vi "(B) Strain Calibration (SubVI).vi"(0 "References":T1, 9 "Strain Input":T3={"cDAQ Chassis"=1, "9237 Slot"=1, "Signals"=[0.10457461685625713, 0.10457461685625713, 0.10457461685625713, 0.10457461685625713]}) -> (6 "Strain OK?":bool, 8 "Strain Values":T2={"Output Values"=[1.9176191262786784, -5.904090522496145, 9.846069970789538, 2.5400406567394125], "Linear Equations"=[["f(x) = 18.337(x)+(0.000)", "18.337", "0.000"], ["f(x) = 22.199(x)+(-8.225)", "22.199", "-8.225"], ["f(x) = 94.154(x)+(0.000)", "94.154", "0.000"], ["f(x) = 24.289(x)+(0.000)", "24.289", "0.000"]], "COF Values"=[0.0, 0.0, 0.0, 0.0], "Signals"=[0.10457461685625713, 0.10457461685625713, 0.10457461685625713, 0.10457461685625713]}, 15 "Calibration Error":errorcluster)   [LabVIEW 2010]
panel:
  in  "Simulation":T4
  in  "Error Input":errorcluster
  in  "Calibration":T5={"Set?"=[FALSE, FALSE, FALSE, FALSE, FALSE, FALSE, FALSE, FALSE], "HI/LO Setpoints"=[10.0, 0.0, 10.0, 0.0, 10.0, 0.0, 10.0, 0.0], "HI/LO Signals"=[1.0, 0.0, 1.0, 0.0, 1.0, 0.0, 1.0, 0.0], "IN/OUT Signals"=[1.0, 0.0, 1.0, 0.0, 1.0, 0.0, 1.0, 0.0]} {"IN/OUT Signals" step=0.001 format="%#_4p"; "HI/LO Signals" step=0.001 format="%#_4p"; "HI/LO Setpoints" step=0.001 format="%#.2p"}
  # "Set\nValues?"
  # "Setpoint\nValues"
  # "Saved\nSignals"
  # "Calibration\nResult"
  # "Ch."
  # "IN"
  # "HI"
  # "0"
  # "LO"
  # "OUT"
  # "IN"
  # "HI"
  # "3"
  # "LO"
  # "OUT"
  # "IN"
  # "HI"
  # "2"
  # "LO"
  # "OUT"
  # "IN"
  # "HI"
  # "1"
  # "LO"
  # "OUT"
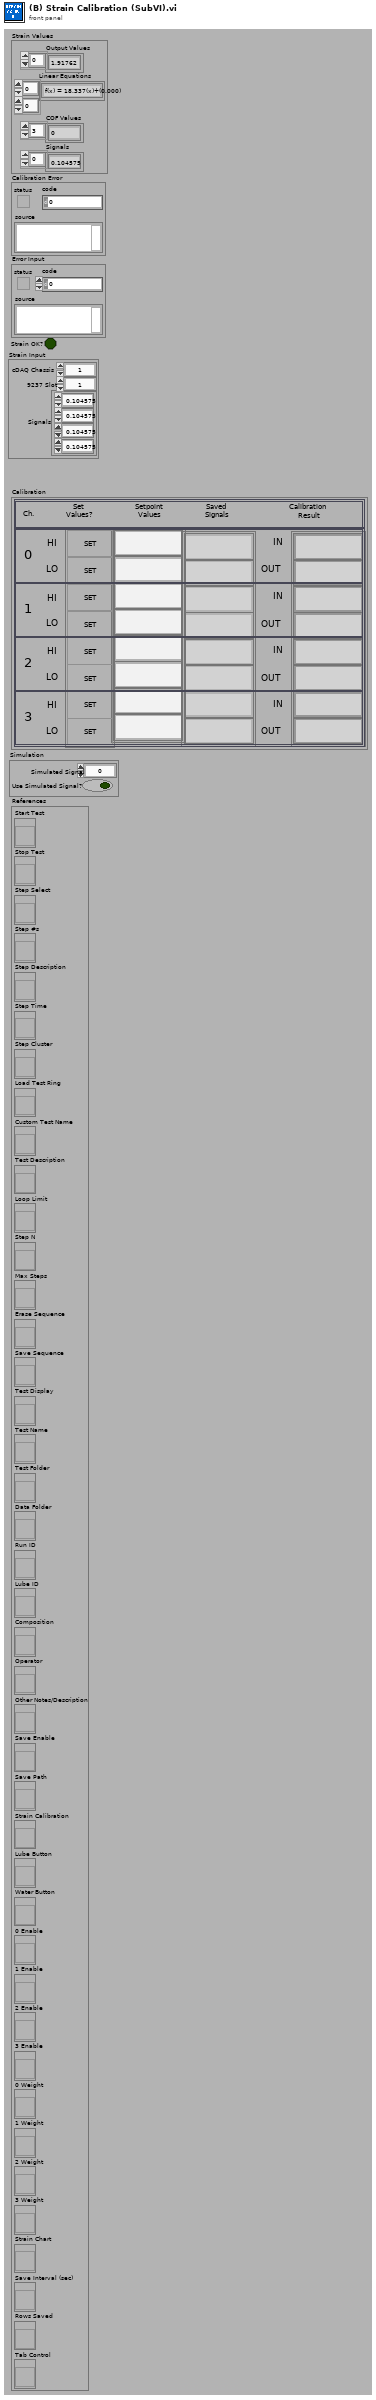
[diagram p1: front panel]
types:
  T1 = cluster{"Start Test":refnum<vi>, "Stop Test":refnum<vi>, "Step Select":refnum<vi>, "Step #s":refnum<vi>, "Step Description":refnum<vi>, "Step Time":refnum<vi>, "Step Cluster":refnum<vi>, "Load Test Ring":refnum<vi>, "Custom Test Name":refnum<vi>, "Test Description":refnum<vi>, "Loop Limit":refnum<vi>, "Step N":refnum<vi>, "Max Steps":refnum<vi>, "Erase Sequence":refnum<vi>, "Save Sequence":refnum<vi>, "Test Display":refnum<vi>, "Test Name":refnum<vi>, "Test Folder":refnum<vi>, "Data Folder":refnum<vi>, "Run ID":refnum<vi>, "Lube ID":refnum<vi>, "Composition":refnum<vi>, "Operator":refnum<vi>, "Other Notes/Description":refnum<vi>, "Save Enable":refnum<vi>, "Save Path":refnum<vi>, "Strain Calibration":refnum<vi>, "Lube Button":refnum<vi>, "Water Button":refnum<vi>, "0 Enable":refnum<vi>, "1 Enable":refnum<vi>, "2 Enable":refnum<vi>, "3 Enable":refnum<vi>, "0 Weight":refnum<vi>, "1 Weight":refnum<vi>, "2 Weight":refnum<vi>, "3 Weight":refnum<vi>, "Strain Chart":refnum<vi>, "Save Interval (sec)":refnum<vi>, "Rows Saved":refnum<vi>, "Tab Control":refnum<vi>}
  T2 = cluster{"Output Values":dbl[], "Linear Equations":string[][], "COF Values":dbl[], "Signals":dbl[]}
  T3 = cluster{"cDAQ Chassis":i32, "9237 Slot":i32, "Signals":dbl[]}
  T4 = cluster{"Use Simulated Signal?":bool, "Simulated Signal":dbl}
  T5 = cluster{"Set?":bool[], "HI/LO Setpoints":dbl[], "HI/LO Signals":dbl[], "IN/OUT Signals":dbl[]}
  T6 = enum16{"open", "replace", "create", "open or create", "replace or create", "replace or create with confirmation"}
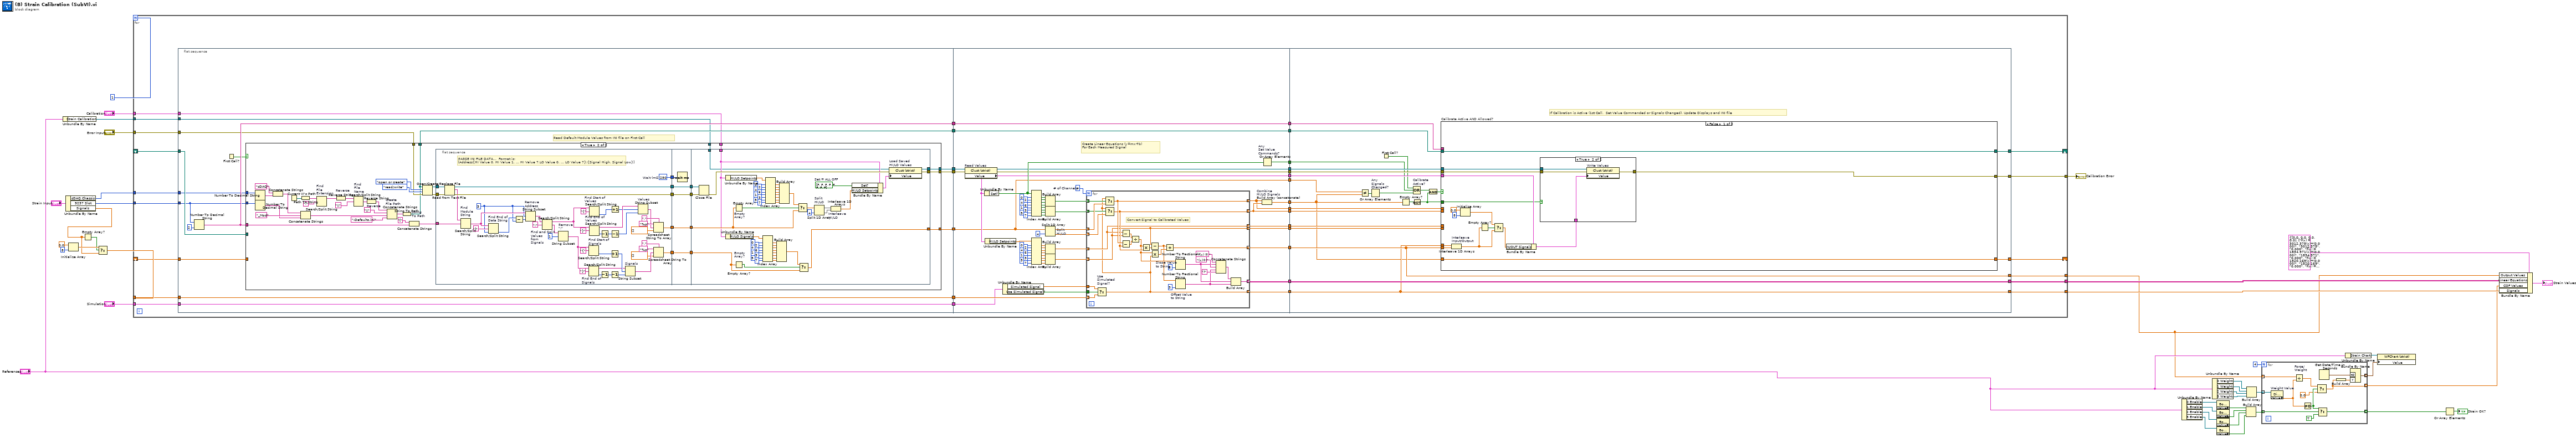
[diagram p0: block diagram]
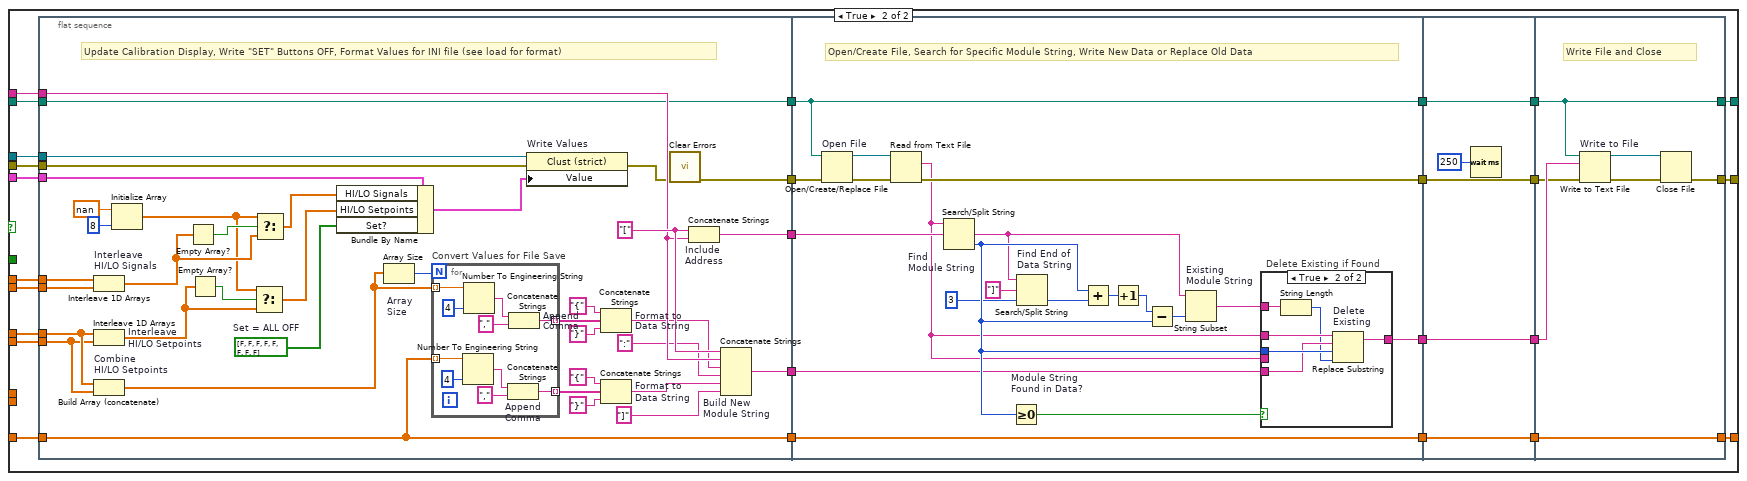
[diagram p4: hidden frame]
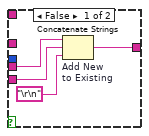
[diagram p5: hidden frame]
diagram:
  n1 = Unbundle By Name("References") -> ("Strain Calibration"=w24:refnum<vi>)
  n2 = Unbundle By Name("Strain Input") -> ("cDAQ Chassis"=w36:i32, "9237 Slot"=w37:i32, "Signals"=w8:dbl[])
  n3 = Initialize Array(0.0, 8) -> (w10:dbl[])
  n4 = Empty Array?(array=w8) -> (empty?=w9:bool)
  n5 = Select(t=w10, s=w9, f=w8) -> (s? t:f=w7:dbl[])
  n6 = for {
    N: 1 -> [_]
    shift-right: [w77] -> _
    shift-left: _ -> [w78]
    tunnel: [w76] -> w13
    shift-right: [w73] -> _
    shift-left: _ -> [w72]
    tunnel: w24 -> [w42]
    tunnel: [w75] -> w1
    tunnel: [w74] -> w27
    tunnel: "Error Input" -> [w67]
    tunnel: [w65] -> w28
    tunnel: "Calibration" -> [w64]
    tunnel: w36 -> [w48]
    tunnel: w37 -> [w47]
    tunnel: "Simulation" -> [w45]
    tunnel: w7 -> [w43]
    n7 = flat-sequence {
      tunnel: [w94] -> w52
      tunnel: [w93] -> w53
      tunnel: [w91] -> w54
      tunnel: [w89] -> w51
      tunnel: [w88] -> w50
      tunnel: [w87] -> w49
      tunnel: [w84] -> w44
      tunnel: w43 -> [w88]
      tunnel: w45 -> [w84]
      tunnel: w47 -> [w82]
      tunnel: w48 -> [w83]
      tunnel: w64 -> [w85]
      tunnel: w67 -> [w86]
      tunnel: w42 -> [w80]
      tunnel: w72 -> [w92]
      tunnel: w78 -> [w90]
      tunnel: [w306] -> w71
      tunnel: [w304] -> w70
      tunnel: [w261] -> w69
      tunnel: [w305] -> w68
      tunnel: [w302] -> w66
      tunnel: [w266] -> w63
      tunnel: [w265] -> w62
      tunnel: [w263] -> w61
      tunnel: [w264] -> w60
      tunnel: [w262] -> w59
      tunnel: [w255] -> w58
      tunnel: [w259] -> w57
      tunnel: [w256] -> w56
      tunnel: [w258] -> w55
      tunnel: w49 -> [w250]
      tunnel: w50 -> [w303]
      tunnel: w51 -> [w260]
      tunnel: w52 -> [w305]
      tunnel: w53 -> [w306]
      tunnel: w54 -> [w255]
      tunnel: [w249] -> w46
      tunnel: w44 -> [w247]
      tunnel: w71 -> [w360]
      tunnel: w70 -> [w340]
      tunnel: w69 -> [w349]
      tunnel: w68 -> [w357]
      tunnel: [w350] -> w75
      tunnel: [w349] -> w74
      tunnel: [w359] -> w76
      tunnel: [w358] -> w77
      tunnel: [w356] -> w73
      tunnel: w66 -> [w355]
      tunnel: [w355] -> w65
      tunnel: w63 -> [w354]
      tunnel: w62 -> [w353]
      tunnel: w61 -> [w352]
      tunnel: w60 -> [w351]
      tunnel: w59 -> [w350]
      tunnel: w58 -> [w347]
      tunnel: w57 -> [w345]
      tunnel: w56 -> [w344]
      tunnel: w55 -> [w346]
      tunnel: w46 -> [w343]
      frame #0 {
        # "Read Default Module Values from INI file on First Call"
        n8 = Number To Decimal String(number=w82, width (-)=i16 2) -> (decimal integer string=w93:string)
        n9 = First Call?() -> (First Call?: T/F=w79:bool)
        n10 = case shown="True" w79 {
          tunnel: w90 -> [w97 _]
          tunnel: [w98 w107] -> w94
          tunnel: w93 -> [_ w134]
          tunnel: w92 -> [w98 _]
          tunnel: [w97 w133] -> w91
          tunnel: [w95 w132] -> w89
          tunnel: w86 -> [w96 w120]
          tunnel: [w96 w119] -> w87
          tunnel: w85 -> [_ w109]
          tunnel: w80 -> [w95 w108]
          tunnel: w83 -> [_ w102]
          tunnel: w82 -> [_ w101]
          frame False {
          }
          frame True {
            n11 = Number To Decimal String(number=w102) -> (decimal integer string=w104:string)  [unwired: 1 in]
            n12 = Number To Decimal String(number=w101) -> (decimal integer string=w105:string)  [unwired: 1 in]
            n13 = Concatenate Strings("cDAQ" ("string"), w104) -> (w103:string)
            n14 = Current VI's Path() -> (path=w128:path)
            n15 = Path To String(path=w128) -> (string=w123:string)
            n16 = Concatenate Strings(w103, "_Mod" ("new task name"), w105) -> (w100:string)
            n17 = Search/Split String "Find\nFile \nExtension"(string=w123, search string/char (-)=".") -> (substring before match=w124:string)  [unwired: 1 in, 2 out]
            n18 = Reverse String "Reverse"(1:w124) -> (0:w125:string)
            n19 = Search/Split String "Find\nFile \nName"(string=w125, search string/char (-)="\\") -> (match + rest of string=w127:string)  [unwired: 1 in, 2 out]
            n20 = Reverse String "Reverse"(1:w127) -> (0:w129:string)
            n21 = Concatenate Strings "Create\nFile Path"(w129, "\\", w100, "-Defaults.ini" ("string")) -> (w131:string)
            n22 = String To Path "String\nTo Path"(string=w131) -> (path=w107:path)
            n23 = Concatenate Strings ("Combine\nCOM Port &\nModule Address")("[" ("string"), w134) -> (w136:string)
            n24 = Open/Create/Replace File(file path (use dialog)=w107, error in=w120, operation (0:open)=T6."open or create", access (0:read/write)=enum16{"read/write", "read-only", "write-only"}."read/write") -> (refnum out=w139:refnum<file>, error out=w138:errorcluster)  [unwired: 3 out]
            n25 = flat-sequence {
              tunnel: [w184] -> w111
              tunnel: [w183] -> w113
              tunnel: w139 -> [w182]
              tunnel: w138 -> [w181]
              tunnel: w136 -> [w175]
              tunnel: [w178] -> w114
              tunnel: [w159] -> w116
              tunnel: [w142] -> w118
              tunnel: w118 -> [w189]
              tunnel: [w189] -> w117
              tunnel: w116 -> [w188]
              tunnel: [w188] -> w115
              tunnel: w114 -> [w185]
              tunnel: w113 -> [w187]
              tunnel: [w187] -> w112
              tunnel: w111 -> [w186]
              tunnel: [w186] -> w110
              tunnel: [w238] -> w133
              tunnel: [w240] -> w132
              tunnel: w117 -> [w218]
              tunnel: w115 -> [w199]
              tunnel: w112 -> [w244]
              tunnel: w110 -> [w243]
              tunnel: [w237] -> w119
              tunnel: w109 -> [w191]
              tunnel: w108 -> [w190]
              frame #0 {
                w141 = 3
                w178 = u32 250  # Wait (mS)
                # "PARSE INI FILE DATA...  Format is:\n[Address{HI Value 0, HI Value 1, ... HI Value 7,LO Value 0, ... LO Value 7}:{Signal High, Signal Low}]"
                n26 = Read from Text File(file (use dialog)=w182, error in=w181) -> (refnum out=w183:refnum<file>, text=w179:string, error out=w184:errorcluster)  [unwired: 1 in, 2 out]
                n27 = Search/Split String "Find\nModule\nString"(string=w179, search string/char (-)=w175) -> (match + rest of string=w174:string)  [unwired: 3 out]
                n28 = Search/Split String "Find End of\nData String"(string=w174, search string/char (-)="]", offset (0)=w141) -> (offset of match=w173:i32)  [unwired: 2 out]
                n29 = Subtract(x=w173, y=w141) -> (x-y=w172:i32)
                n30 = String Subset "Remove\nAddress"(string=w174, offset (0)=w141, length (rest)=w172) -> (substring=w171:string)
                n31 = Search/Split String "Find and Split \nValues\nfrom \nSignals"(string=w171, search string/char (-)=":") -> (substring before match=w170:string, match + rest of string=w144:string)  [unwired: 2 out]
                n32 = String Subset "Remove\n\":\""(string=w144, offset (0)=1) -> (substring=w143:string)  [unwired: 1 out]
                n33 = Search/Split String "Find Start of\nSignals"(string=w143, search string/char (-)="{") -> (offset of match=w146:i32)  [unwired: 3 out]
                n34 = Search/Split String "Find End of\nSignals"(string=w143, search string/char (-)="}") -> (substring before match=w151:string, offset of match=w152:i32)  [unwired: 2 out]
                n35 = Search/Split String "Find Start of\nValues"(string=w170, search string/char (-)="{") -> (offset of match=w166:i32)  [unwired: 3 out]
                n36 = Search/Split String "Find End of\nValues"(string=w170, search string/char (-)="}") -> (substring before match=w168:string, offset of match=w167:i32)  [unwired: 2 out]
                n37 = Decrement(x=w167) -> (x-1=w148:i32)
                n38 = Decrement(x=w152) -> (x-1=w147:i32)
                n39 = Increment(x=w146) -> (x+1=w153:i32)
                n40 = Decrement(x=w147) -> (x-1=w154:i32)
                n41 = Increment(x=w166) -> (x+1=w165:i32)
                n42 = Decrement(x=w148) -> (x-1=w164:i32)
                n43 = String Subset "Signals"(string=w151, offset (0)=w153, length (rest)=w154) -> (substring=w158:string)
                n44 = String Subset "Values"(string=w168, offset (0)=w165, length (rest)=w164) -> (substring=w160:string)
                n45 = Spreadsheet String To Array(delimiter (Tab)=",", format string="%p", spreadsheet string=w160, array type (2D Dbl)=dbl[] [] ("array")) -> (array=w159:dbl[])
                n46 = Spreadsheet String To Array(delimiter (Tab)=",", format string="%p", spreadsheet string=w158, array type (2D Dbl)=dbl[] [] ("array")) -> (array=w142:dbl[])
              }
              frame #1 {
                n47 = Wait (ms)(milliseconds to wait=w185) -> ()  [unwired: 1 out]
              }
              frame #2 {
                w192 = bool[] [FALSE, FALSE, FALSE, FALSE, FALSE, FALSE, FALSE, FALSE]  # Set = ALL OFF
                n48 = Close File(refnum=w244, error in=w243) -> (error out=w236:errorcluster)  [unwired: 1 out]
                n49 = Unbundle By Name(w191) -> ("HI/LO Signals"=w193:dbl[])
                n50 = Unbundle By Name(w191) -> ("HI/LO Setpoints"=w201:dbl[])
                n51 = Empty Array? "Empty\nArray?"(array=w199) -> (empty?=w241:bool)
                n52 = Empty Array? "Empty\nArray?"(array=w218) -> (empty?=w242:bool)
                n53 = Index Array(array=w193, index #1=0, index #2=2, index #3=4, index #4=6, index #5=1, index #6=3, index #7=5, index #8=7) -> (element #1=w228:dbl, element #2=w227:dbl, element #3=w226:dbl, element #4=w225:dbl, element #5=w223:dbl, element #6=w222:dbl, element #7=w221:dbl, element #8=w220:dbl)
                n54 = Index Array(array=w201, index #1=0, index #2=2, index #3=4, index #4=6, index #5=1, index #6=3, index #7=5, index #8=7) -> (element #1=w210:dbl, element #2=w209:dbl, element #3=w208:dbl, element #4=w207:dbl, element #5=w205:dbl, element #6=w204:dbl, element #7=w203:dbl, element #8=w202:dbl)
                n55 = Build Array(w228, w227, w226, w225, w223, w222, w221, w220) -> (w219:dbl[])
                n56 = Build Array(w210, w209, w208, w207, w205, w204, w203, w202) -> (w200:dbl[])
                n57 = Select(t=w200, s=w241, f=w199) -> (s? t:f=w198:dbl[])
                n58 = Select(t=w219, s=w242, f=w218) -> (s? t:f=w238:dbl[])
                n59 = Split 1D Array "Split\nHI/LO"(array=w198, index=4) -> (first subarray=w196:dbl[], second subarray=w195:dbl[])
                n60 = Interleave 1D Arrays "Interleave\nHI/LO"(w196, w195) -> (w194:dbl[])
                n61 = Bundle By Name(cluster=w191, "Set?"=w192, "HI/LO Setpoints"=w194) -> (w239:T5)
                n62 = property on="Load Saved\nHI/LO Values" class="Clust (strict)"(reference=w190, error in=w236, "Value"=w239) -> (reference out=w240:refnum<vi>, error out=w237:errorcluster)
              }
            }
          }
        }
      }
      frame #1 {
        w267 = 4  # # of Channels
        # "Create Linear Equations (y=mx+b)\nFor Each Measured Signal"
        n63 = property on="Read Values" class="Clust (strict)"(reference=w260, error in=w250) -> (reference out=w259:refnum<vi>, error out=w258:errorcluster, "Value"=w256:T5)
        n64 = Unbundle By Name(w256) -> ("Set?"=w307:bool[])
        n65 = Unbundle By Name(w256) -> ("HI/LO Setpoints"=w257:dbl[])
        n66 = Unbundle By Name(w247) -> ("Simulated Signal"=w246:dbl, "Use Simulated Signal?"=w245:bool)
        n67 = Index Array(array=w307, index #1=0, index #2=2, index #3=4, index #4=6, index #5=1, index #6=3, index #7=5, index #8=7) -> (element #1=w278:bool, element #2=w277:bool, element #3=w276:bool, element #4=w275:bool, element #5=w274:bool, element #6=w273:bool, element #7=w272:bool, element #8=w252:bool)
        n68 = Index Array(array=w257, index #1=0, index #2=2, index #3=4, index #4=6, index #5=1, index #6=3, index #7=5, index #8=7) -> (element #1=w293:dbl, element #2=w292:dbl, element #3=w291:dbl, element #4=w290:dbl, element #5=w289:dbl, element #6=w288:dbl, element #7=w287:dbl, element #8=w286:dbl)
        n69 = Build Array(w278, w277, w276, w275) -> (w271:bool[])
        n70 = Build Array(w274, w273, w272, w252) -> (w270:bool[])
        n71 = Split 1D Array "Split\nHI/LO"(array=w255, index=4) -> (first subarray=w254:dbl[], second subarray=w253:dbl[])
        n72 = Build Array(w293, w292, w291, w290) -> (w269:dbl[])
        n73 = Build Array(w289, w288, w287, w286) -> (w268:dbl[])
        n74 = for {
          N: w267 -> [_]
          tunnel: [w328] -> w263 mode=indexing
          tunnel: [w327] -> w264 mode=indexing
          tunnel: w254 -> [w331] mode=indexing
          tunnel: w253 -> [w330] mode=indexing
          tunnel: [w329] -> w262 mode=indexing
          tunnel: [w308] -> w261 mode=indexing
          tunnel: [w310] -> w266 mode=indexing
          tunnel: [w309] -> w265 mode=indexing
          tunnel: w303 -> [w326] mode=indexing
          tunnel: [w316] -> w302 mode=indexing
          tunnel: w246 -> [w314]
          tunnel: w245 -> [w313]
          tunnel: w271 -> [w312] mode=indexing
          tunnel: w270 -> [w311] mode=indexing
          tunnel: w269 -> [w310] mode=indexing
          tunnel: w268 -> [w309] mode=indexing
          # "Convert Signal to Calibrated Values"
          n75 = Select "Use\nSimulated\nSignal?"(t=w314, s=w313, f=w326) -> (s? t:f=w308:dbl)
          n76 = Select ("Set HI?")(t=w308, s=w312, f=w331) -> (s? t:f=w328:dbl)
          n77 = Select ("Set LO?")(t=w308, s=w311, f=w330) -> (s? t:f=w327:dbl)
          n78 = Subtract(x=w310, y=w309) -> (x-y=w332:dbl)
          n79 = Subtract(x=w328, y=w327) -> (x-y=w333:dbl)
          n80 = Divide(x=w332, y=w333) -> (x/y=w320:dbl)
          n81 = Multiply(x=w320, y=w327) -> (x*y=w334:dbl)
          n82 = Subtract(x=w309, y=w334) -> (x-y=w319:dbl)
          n83 = Multiply(x=w320, y=w308) -> (x*y=w335:dbl)
          n84 = Add(x=w319, y=w335) -> (x+y=w329:dbl)
          n85 = Number To Fractional String "Slope Value\nto String"(number=w320, precision (6)=i16 3) -> (F-format string=w318:string)  [unwired: 2 in]
          n86 = Number To Fractional String "Offset Value\nto String"(number=w319, precision (6)=i16 3) -> (F-format string=w317:string)  [unwired: 2 in]
          n87 = Concatenate Strings("f(x) = " ("string"), w318, "(x)+(" ("string"), w317, ")" ("string")) -> (w315:string)
          n88 = Build Array(w315, w318, w317) -> (w316:string[])
        }
        n89 = Build Array (concatenate) "Combine\nHI/LO Signals"(w263, w264) -> (w304:dbl[])
        n90 = Or Array Elements "Any\nSet Value\nCommands?"(Boolean array=w307) -> (logical OR=w249:bool)
      }
      frame #2 {
        # "If Calibration is Active (1st Call,  Set Value Commanded or Signals Changed), Update Displays and INI file"
        n91 = Not Equal?(x=w347, y=w340) -> (x != y?=w348:bool[])
        n92 = Or Array Elements "Any\nSignals\nChanged?"(Boolean array=w348) -> (logical OR=w341:bool)
        n93 = First Call?() -> (First Call?: T/F=w342:bool)
        n94 = Empty Array?(array=w340) -> (empty?=w339:bool)
        n95 = Not(x=w339) -> (.not. x?=w336:bool)
        n96 = Compound Arithmetic op=OR "Calibrate\nActive?"(w342, w343, w341) -> (w338:bool)
        n97 = And(x=w338, y=w336) -> (x .and. y?=w337:bool)
        n98 = case "Calibrate Active AND Allowed?" shown="False" w337 {
          tunnel: w357 -> [w376 w403]
          tunnel: w360 -> [_ w407]
          tunnel: w340 -> [w375 w406]
          tunnel: [w373 w405] -> w359
          tunnel: [w375 w404] -> w358
          tunnel: [w376 w402] -> w356
          tunnel: w354 -> [_ w401]
          tunnel: w353 -> [_ w400]
          tunnel: w352 -> [_ w399]
          tunnel: w351 -> [_ w398]
          tunnel: w350 -> [w371 _]
          tunnel: w349 -> [w372 _]
          tunnel: w344 -> [w370 w384]
          tunnel: w346 -> [w369 w383]
          tunnel: w345 -> [w368 w382]
          tunnel: w336 -> [w361 _]
          frame False {
            n99 = Interleave 1D Arrays "Interleave\nInput/Output"(w372, w371) -> (w364:dbl[])
            n100 = Initialize Array(0.0, 8) -> (w365:dbl[])
            n101 = Empty Array?(array=w364) -> (empty?=w363:bool)
            n102 = Select(t=w365, s=w363, f=w364) -> (s? t:f=w362:dbl[])
            n103 = Bundle By Name(cluster=w370, "IN/OUT Signals"=w362) -> (w374:T5)
            n104 = case shown="True" w361 {
              tunnel: w374 -> [_ w381]
              tunnel: [w377 w380] -> w373
              tunnel: w369 -> [w377 w379]
              tunnel: w368 -> [_ w378]
              frame False {
              }
              frame True {
                n105 = property on="Write Values" class="Clust (strict)"(reference=w378, error in=w379, "Value"=w381) -> (error out=w380:errorcluster)  [unwired: 1 out]
              }
            }
          }
          frame True {
            n106 = flat-sequence {
              tunnel: [w421] -> w389
              tunnel: [w439] -> w388
              tunnel: [w438] -> w387
              tunnel: [w437] -> w386
              tunnel: [w436] -> w385
              tunnel: w398 -> [w424]
              tunnel: w399 -> [w425]
              tunnel: w400 -> [w422]
              tunnel: w401 -> [w423]
              tunnel: w403 -> [w436]
              tunnel: w406 -> [w438]
              tunnel: w407 -> [w440]
              tunnel: w384 -> [w420]
              tunnel: w383 -> [w419]
              tunnel: w382 -> [w418]
              tunnel: [w469] -> w397
              tunnel: [w470] -> w395
              tunnel: [w468] -> w393
              tunnel: [w462] -> w391
              tunnel: w385 -> [w462]
              tunnel: w386 -> [w467]
              tunnel: w387 -> [w468]
              tunnel: w388 -> [w463]
              tunnel: w389 -> [w456]
              tunnel: w397 -> [w490]
              tunnel: [w490] -> w396
              tunnel: w395 -> [w489]
              tunnel: [w489] -> w394
              tunnel: w393 -> [w488]
              tunnel: [w488] -> w392
              tunnel: w391 -> [w487]
              tunnel: [w487] -> w390
              tunnel: [w495] -> w405
              tunnel: [w494] -> w404
              tunnel: [w493] -> w402
              tunnel: w390 -> [w493]
              tunnel: w392 -> [w494]
              tunnel: w394 -> [w492]
              tunnel: w396 -> [w491]
              frame #0 {
                w417 = bool[] [FALSE, FALSE, FALSE, FALSE, FALSE, FALSE, FALSE, FALSE]  # Set = ALL OFF
                w442 = "[" ("string")
                # "Update Calibration Display, Write \"SET\" Buttons OFF, Format Values for INI file (see load for format)"
                n107 = Interleave 1D Arrays "Interleave\nHI/LO Signals"(w425, w424) -> (w412:dbl[])
                n108 = Interleave 1D Arrays "Interleave\nHI/LO Setpoints"(w423, w422) -> (w409:dbl[])
                n109 = Build Array (concatenate) "Combine\nHI/LO Setpoints"(w423, w422) -> (w435:dbl[])
                n110 = Initialize Array(nan, 8) -> (w411:dbl[])
                n111 = Empty Array?(array=w412) -> (empty?=w414:bool)
                n112 = Empty Array?(array=w409) -> (empty?=w408:bool)
                n113 = Select(t=w411, s=w408, f=w409) -> (s? t:f=w410:dbl[])
                n114 = Select(t=w411, s=w414, f=w412) -> (s? t:f=w413:dbl[])
                n115 = Bundle By Name(cluster=w420, "HI/LO Signals"=w413, "HI/LO Setpoints"=w410, "Set?"=w417) -> (w426:T5)
                n116 = Array Size "Array\nSize"(array=w435) -> (size(s)=w441:i32)
                n117 = for "Convert Values for File Save" {
                  N: w441 -> [_]
                  tunnel: w438 -> [w455] mode=indexing
                  tunnel: [w451] -> w444 mode=indexing
                  tunnel: w435 -> [w447] mode=indexing
                  tunnel: [w446] -> w432 mode=indexing
                  n118 = Number To Engineering String(2:i16 4 ("precision (6)"), 4:w455) -> (0:w453:string)  [unwired: 2 in]
                  n119 = Number To Engineering String(2:i16 4 ("precision (6)"), 4:w447) -> (0:w449:string)  [unwired: 2 in]
                  n120 = Concatenate Strings "Append\nComma"(w453, ",") -> (w451:string)
                  n121 = Concatenate Strings "Append\nComma"(w449, ",") -> (w446:string)
                }
                n122 = property on="Write Values" class="Clust (strict)"(reference=w418, error in=w419, "Value"=w426) -> (error out=w427:errorcluster)  [unwired: 1 out]
                n123 = Concatenate Strings "Format to\nData String"("{", w432, "}") -> (w431:string)
                n124 = Concatenate Strings "Format to\nData String"("{", w444, "}") -> (w429:string)
                n125 = call <vilib>:"Clear Errors.vi"("error in (no error)"=w427) -> ("error out"=w421:errorcluster)  [unwired: 6 out]
                n126 = Concatenate Strings "Include\nAddress"(w442, w440) -> (w437:string)
                n127 = Concatenate Strings "Build New\nModule String"(w442, w440, w431, ":" ("string"), w429, "]" ("string")) -> (w439:string)
              }
              frame #1 {
                # "Open/Create File, Search for Specific Module String, Write New Data or Replace Old Data"
                n128 = Open/Create/Replace File "Open File"(file path (use dialog)=w462, error in=w456) -> (refnum out=w458:refnum<file>, error out=w457:errorcluster)  [unwired: 5 out]
                n129 = Read from Text File(file (use dialog)=w458, error in=w457) -> (text=w459:string, error out=w469:errorcluster)  [unwired: 1 in, 3 out]
                n130 = Search/Split String "Find\nModule String"(string=w459, search string/char (-)=w467) -> (match + rest of string=w472:string, offset of match=w475:i32)  [unwired: 2 out]
                n131 = Greater Or Equal To 0? "Module String\nFound in Data?"(x=w475) -> (x >= 0?=w474:bool)
                n132 = Search/Split String "Find End of\nData String"(string=w472, search string/char (-)="]", offset (0)=3) -> (offset of match=w465:i32)  [unwired: 2 out]
                n133 = Add(x=w475, y=w465) -> (x+y=w464:i32)
                n134 = Increment(x=w464) -> (x+1=w466:i32)
                n135 = Subtract(x=w466, y=w475) -> (x-y=w473:i32)
                n136 = String Subset "Existing\nModule String"(string=w472, length (rest)=w473) -> (substring=w461:string)  [unwired: 1 out]
                n137 = case "Delete Existing if Found" shown="True" w474 {
                  tunnel: w459 -> [_ w485]
                  tunnel: [w477 w484] -> w470
                  tunnel: w475 -> [_ w483]
                  tunnel: w463 -> [w478 w482]
                  tunnel: w461 -> [_ w480]
                  tunnel: w459 -> [w479 _]
                  frame False {
                    n138 = Concatenate Strings "Add New\nto Existing"(w479, w478, "\r\n") -> (w477:string)
                  }
                  frame True {
                    n139 = String Length(string=w480) -> (length=w481:i32)
                    n140 = Replace Substring "Delete\nExisting"(2:w481, 3:w483, 4:w482, 5:w485) -> (1:w484:string)  [unwired: 1 out]
                  }
                }
              }
              frame #2 {
                n141 = Wait (ms)(milliseconds to wait=u32 250) -> ()  [unwired: 1 out]
              }
              frame #3 {
                # "Write File and Close"
                n142 = Write to Text File "Write to File"(file (use dialog)=w493, text=w492, error in=w491) -> (refnum out=w497:refnum<file>, error out=w496:errorcluster)  [unwired: 2 out]
                n143 = Close File(refnum=w497, error in=w496) -> (error out=w495:errorcluster)  [unwired: 1 out]
              }
            }
          }
        }
      }
    }
  }
  "Calibration Error" <- w13
  n144 = Unbundle By Name("References") -> ("0 Enable"=w23:refnum<vi>, "1 Enable"=w22:refnum<vi>, "2 Enable"=w21:refnum<vi>, "3 Enable"=w20:refnum<vi>)
  n145 = Unbundle By Name("References") -> ("0 Weight"=w35:refnum<vi>, "1 Weight"=w34:refnum<vi>, "2 Weight"=w33:refnum<vi>, "3 Weight"=w32:refnum<vi>)
  n146 = property class="Bool (strict)"(reference=w23) -> ("Value"=w19:bool)  [unwired: 1 in, 2 out]
  n147 = property class="Bool (strict)"(reference=w22) -> ("Value"=w18:bool)  [unwired: 1 in, 2 out]
  n148 = property class="Bool (strict)"(reference=w21) -> ("Value"=w17:bool)  [unwired: 1 in, 2 out]
  n149 = property class="Bool (strict)"(reference=w20) -> ("Value"=w16:bool)  [unwired: 1 in, 2 out]
  n150 = Build Array(w19, w18, w17, w16) -> (w4:bool[])
  n151 = Build Array(w35, w34, w33, w32) -> (w5:refnum<vi>[])
  n152 = for {
    N: 4 -> [_]
    tunnel: w5 -> [w505] mode=indexing
    tunnel: w1 -> [w510] mode=indexing
    tunnel: [w499] -> w26 mode=indexing
    tunnel: [w507] -> w31 mode=indexing
    tunnel: w4 -> [w506] mode=indexing
    tunnel: [w503] -> w3 mode=indexing
    n153 = property on="Weight Value" class="DigNum (strict)"(reference=w505) -> ("Value"=w509:dbl)  [unwired: 1 in, 2 out]
    n154 = Divide "Force/\nWeight"(x=w510, y=w509) -> (x/y=w500:dbl)
    n155 = Not Equal To 0?(x=w509) -> (x != 0?=w502:bool)
    n156 = Select(t=w500, s=w502, f=0.0) -> (s? t:f=w499:dbl)
    n157 = Select(t=w502, s=w506, f=TRUE) -> (s? t:f=w507:bool)
    n158 = Get Date/Time In Seconds() -> (seconds since 1Jan1904=w498:timestamp)
    n159 = Build Array(w499) -> (w504:dbl[])
    n160 = Bundle By Name("t0"=w498, "Y"=w504) -> (w503:waveform(dbl))  [unwired: 1 in]
  }
  n161 = Unbundle By Name("References") -> ("Strain Chart"=w2:refnum<vi>)
  n162 = property class="WFChart (strict)"(reference=w2, "Value"=w3) -> ()  [unwired: 1 in, 2 out]
  n163 = Or Array Elements(Boolean array=w31) -> (logical OR=→"Strain OK?":bool)
  n164 = Bundle By Name(cluster=T2 {"Output Values"=[0.0, 0.0, 0.0, 0.0], "Linear Equations"=[["f(x) = 3012.375(x)+(0.000)", "3012.375", "0.000"], ["f(x) = 1834.971(x)+(0.000)", "1834.971", "0.000"], ["f(x) = 1520.169(x)+(0.000)", "1520.169", "0.000"], ["f(x) = 657.495(x)+(0.000)", "657.495", "0.000"]], "COF Values"=[0.0, 0.0, 0.0, 0.0], "Signals"=[0.0, 0.0, 0.0, 0.0]} ("Strain Cluster"), "Output Values"=w1, "Linear Equations"=w28, "COF Values"=w26, "Signals"=w27) -> (→"Strain Values":T2)
